vi "thermometer.vi"(10 "y":dbl, 11 "x":dbl) -> (3 "Numeric":dbl)   [LabVIEW 2014]
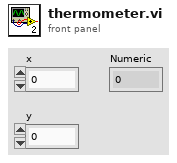
[diagram p1: front panel]
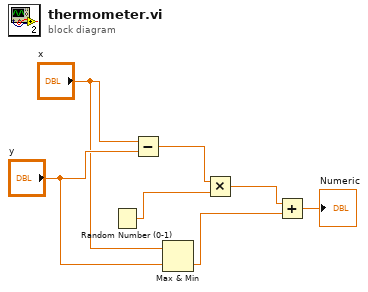
[diagram p0: block diagram]
diagram:
  n1 = Random Number (0-1)() -> (number: 0 to 1=w2:dbl)
  n2 = Subtract(x="x", y="y") -> (x-y=w1:dbl)
  n3 = Max & Min(x="x", y="y") -> (min(x,y)=w4:dbl)  [unwired: 1 out]
  n4 = Multiply(x=w1, y=w2) -> (x*y=w3:dbl)
  n5 = Add(x=w3, y=w4) -> (x+y=→"Numeric":dbl)
